vi "To CSV File.vi"(8 "error in (no error)":errorcluster, 9 "Path":path, 10 "engine configuration":refnum<class "engine configuration.lvclass">, 11 "tag select module editor node in":refnum<class "tag select module editor node.lvclass">) -> (0 "error out":errorcluster, 3 "tag select module editor node out":refnum<class "tag select module editor node.lvclass">)   [LabVIEW 2015, in "tag select module editor node.lvclass"]
uses:
  tag select module editor node.lvclass
  <vilib>/NI/Module Execution Interface/Engine Configuration/engine configuration.lvclass
  module/configuration/tag select module configuration.lvclass
  <vilib>/NI/Configuration Framework/serializable configuration/NISE_CEF_serializable configuration.lvclass/NISE_CEF_serializable configuration.ctl
  module/configuration/tag select module configuration.lvclass/tag select module configuration.ctl
  <vilib>/NI/Tag Bus/tag/tag descriptor.lvclass/tag descriptor.ctl
  module/configuration/Read tag select.vi
  <vilib>/Utility/LVClass/Get LV Class Name.vi
  <vilib>/NI/Configuration Framework/error generator/NISE_error generator.vi
  <vilib>/NI/Tag Bus Module Framework/channel/TBM channel.lvclass
  <vilib>/NI/Configuration Framework/serializable configuration/NISE_CEF_serializable configuration.lvclass
  <vilib>/NI/Tag Bus/tag/tag descriptor.lvclass
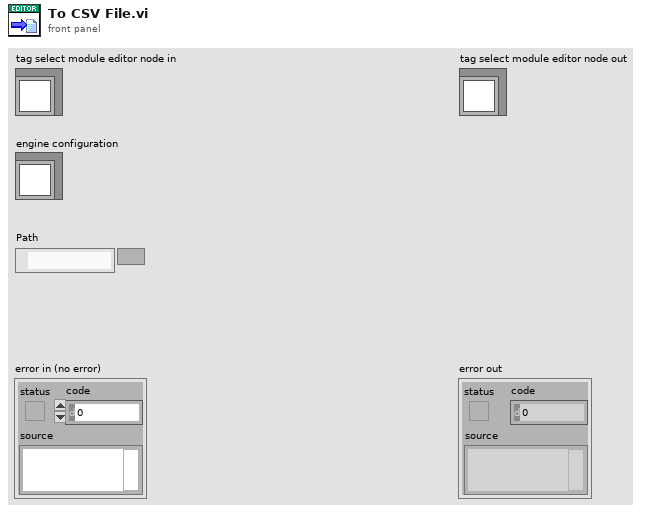
[diagram p1: front panel]
types:
  T1 = typedef "tag select module configuration.lvclass/tag select configuration.ctl" = cluster{"tag select name":string, "data type":T2, "output":refnum<class "TBM channel.lvclass">, "select":refnum<class "TBM channel.lvclass">, "input channels":refnum<class "TBM channel.lvclass">[]}
  T2 = typedef "tag bus.lvlib/tag descriptor.lvclass/Data Type.ctl" = enum16{"Double", "Single", "I64", "I32", "I16", "I8", "U64", "U32", "U16", "U8", "Boolean", "String", "Array of Double", "Array of Single", "Array of I64", "Array of I32", "Array of I16", "Array of I8", "Array of U64", "Array of U32", "Array of U16", "Array of U8", "Array of Boolean", "Array of String"}
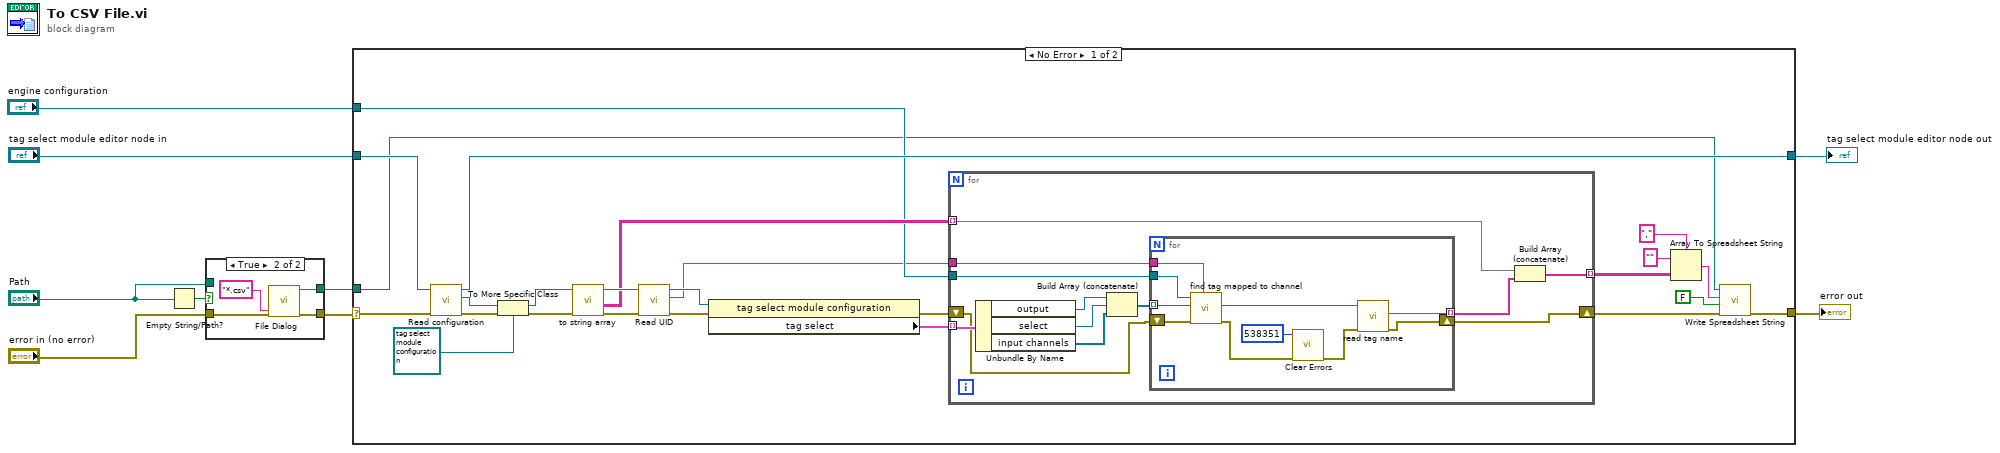
[diagram p0: block diagram]
diagram:
  n1 = Empty String/Path?(string/path="Path") -> (empty?=w9:bool)
  n2 = case shown="True" w9 {
    tunnel: "error in (no error)" -> [w10 w14]
    tunnel: [w10 w13] -> w6
    tunnel: [w11 w12] -> w5
    tunnel: "Path" -> [w11 _]
    frame False {
    }
    frame True {
      n3 = call "File Dialog"("error in"=w14, "pattern (all files)"="*.csv") -> ("selected path"=w12:path, "error out"=w13:errorcluster)  [unwired: 10 in, 2 out]
    }
  }
  n4 = case shown="No Error" w6 {
    selector: w6 -> [w39 w63]
    tunnel: w5 -> [w16 _]
    tunnel: "tag select module editor node in" -> [w40 w64]
    tunnel: [w36 w64] -> w3
    tunnel: "engine configuration" -> [w26 _]
    tunnel: [w17 w63] -> w1
    frame No Error {
      n5 = call-dynamic "Read configuration.vi"("error in"=w39, "tag select module editor node in"=w40) -> ("error out"=w38:errorcluster, "configuration"=w37:refnum<class "NISE_CEF_serializable configuration.lvclass">, "tag select module editor node out"=w36:refnum<class "tag select module editor node.lvclass">)  [unwired: 7 in]
      n6 = To More Specific Class(target class=refnum<class "tag select module configuration.lvclass"> refnum ("tag select module configuration"), reference=w37, error in=w38) -> (specific class reference=w33:refnum<class "tag select module configuration.lvclass">, error out=w34:errorcluster)
      n7 = call-dynamic "to string array.vi"("error in (no error)"=w34, "module configuration in"=w33) -> ("error out"=w32:errorcluster, "Array"=w27:string[][], "module configuration out"=w31:refnum<class "tag select module configuration.lvclass">)  [unwired: 6 in, 1 out]
      n8 = call <vilib>:"Read UID.vi"("error in"=w32, "configuration in"=w31) -> ("error out"=w29:errorcluster, "instance id"=w25:string, "configuration out"=w30:refnum<class "tag select module configuration.lvclass">)  [unwired: 7 in]
      n9 = property class="tag select module configuration"(reference=w30, error in=w29) -> (error out=w24:errorcluster, "tag select"=w28:T1[])  [unwired: 1 out]
      n10 = for {
        tunnel: w28 -> [w50] mode=indexing
        tunnel: w27 -> [w52] mode=indexing
        tunnel: [w51] -> w19 mode=indexing
        tunnel: w26 -> [w44]
        tunnel: w25 -> [w43]
        shift-right: [w42] -> w18
        shift-left: w24 -> [w41]
        n11 = Unbundle By Name(w50) -> ("output"=w48:refnum<class "TBM channel.lvclass">, "select"=w47:refnum<class "TBM channel.lvclass">, "input channels"=w49:refnum<class "TBM channel.lvclass">[])
        n12 = Build Array (concatenate)(w48, w47, w49) -> (w46:refnum<class "TBM channel.lvclass">[])
        n13 = for {
          tunnel: w46 -> [w62] mode=indexing
          tunnel: [w60] -> w45 mode=indexing
          tunnel: w44 -> [w59]
          tunnel: w43 -> [w58]
          shift-right: [w56] -> w42
          shift-left: w41 -> [w57]
          n14 = call <vilib>:"find tag mapped to channel.vi"("owner"=w58, "error in"=w57, "channel"=w62, "engine configuration in"=w59) -> ("error out"=w54:errorcluster, "tag"=w61:refnum<class "tag descriptor.lvclass">)  [unwired: 5 in, 1 out]
          n15 = call <vilib>:"Clear Errors.vi"("error in (no error)"=w54, "specific error code to clear (0: all)"=538351) -> ("error out"=w53:errorcluster)  [unwired: 4 in, 1 out]
          n16 = call <vilib>:"read tag name.vi"("error in"=w53, "system tag in"=w61) -> ("error out"=w56:errorcluster, "name"=w60:string)  [unwired: 7 in, 1 out]
        }
        n17 = Build Array (concatenate)(w52, w45) -> (w51:string[])
      }
      n18 = Array To Spreadsheet String(delimiter (Tab)=",", array=w19, 3:"" ("format string")) -> (spreadsheet string=w23:string)
      n19 = call <vilib>:"Write Spreadsheet String.vi"("error in"=w18, "append to file? (new file:F)"=FALSE, "spreadsheet string"=w23, "file path (dialog if empty)"=w16) -> ("error out"=w17:errorcluster)  [unwired: 6 in, 1 out]
    }
    frame Error {
    }
  }
  "error out" <- w1
  "tag select module editor node out" <- w3
